vi "TestOsc.vi"() -> ()   [LabVIEW 2014]
panel:
  in  "stop":bool
  out "Waveform Chart":dbl(graph)
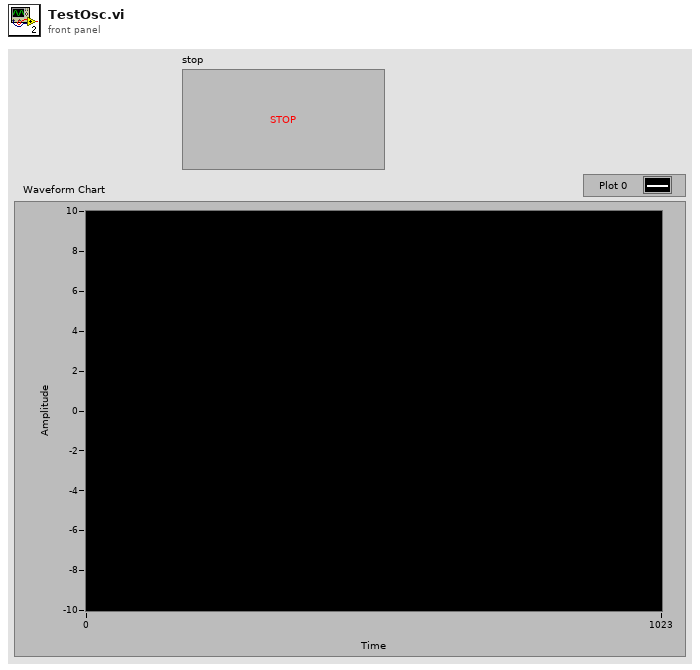
[diagram p1: front panel]
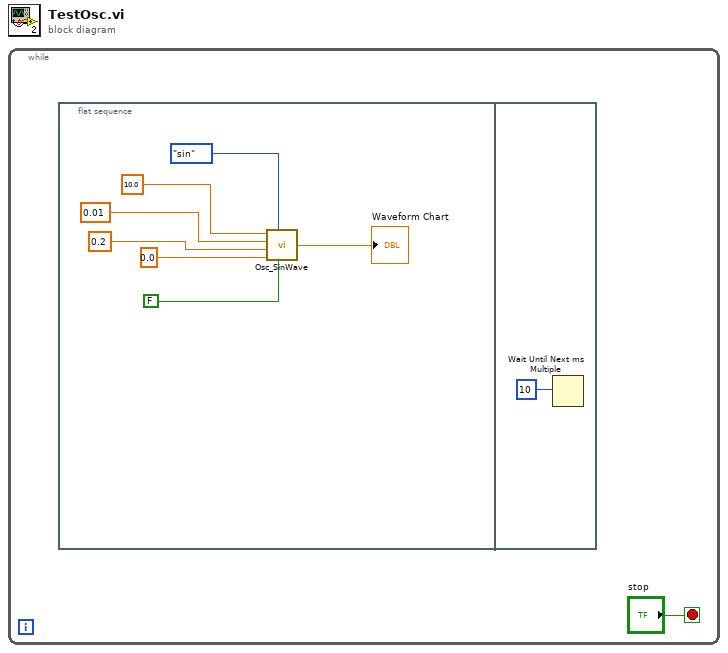
[diagram p0: block diagram]
diagram:
  n1 = while {
    stop <- "stop" stop-if-true
    n2 = flat-sequence {
      frame #0 {
        n3 = call "Osc_SinWave.vi"("Reset"=FALSE, "WaveType"=enum16{"sin", "cos"}."sin", "Phase"=0.0, "step_t"=0.2, "Frequency/Hz"=0.01, "Amplitude"=10.0) -> ("Wave"=→"Waveform Chart":dbl)
      }
      frame #1 {
        n4 = Wait Until Next ms Multiple(millisecond multiple=u32 10 ("milliseconds to wait")) -> ()  [unwired: 1 out]
      }
    }
  }
